vi "fgv_AO_daqmx.vi"(7 "cmd":T1=enum."init", 8 "error in":errorcluster, 11 "level":bool) -> (0 "error out":errorcluster)   [LabVIEW 2019]
uses:
  _ctrl/init-w-close.ctl
  _ctrl/rw.ctl
  SubVIs/common/cmd_err.ctl
  <vilib>/DAQmx/write.llb/DAQmx Write (Analog Wfm 1Chan NSamp).vi
  SubVIs/common/Glob_Ref.vi
  <vilib>/DAQmx/create/channels.llb/DAQmx Create Channel (AO-Voltage-Basic).vi
  <vilib>/DAQmx/configure/timing.llb/DAQmx Timing (Sample Clock).vi
  <vilib>/DAQmx/miscellaneous.llb/DAQmx Fill In Error Info.vi
  Durability/common/Global_params.vi
panel:
  out "task out":refnum<k21>
  out "Waveform Graph":waveform(dbl)(graph)
  out "sample mode":i32(ring)=10178 items=["유한 샘플"=10178, "연속 샘플"=10123, "하드웨어 타이밍에 의한 단일 포인트"=12522]
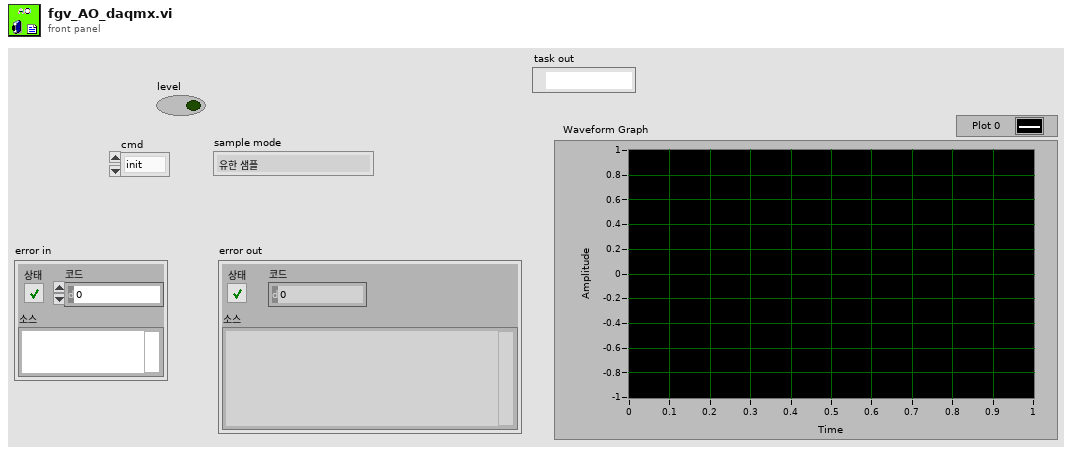
[diagram p1: front panel]
types:
  T1 = typedef "init-w-close.ctl" = enum16{"open", "init", "write", "close"}
  T2 = enum16{"DL950", "BP4610", "DSP1500", "cDAQ-AI", "cDAQ-AO", "cDAQ-DO"}
  T3 = typedef "cmd_err.ctl" = enum16{"close", "open", "default"}
  T4 = typedef "rw.ctl" = enum16{"read", "write"}
  T5 = typedef "cDAQ-9269 Config.ctl" = cluster{"Ch":tag, "Max V":dbl, "Min V":dbl, " Rate":dbl, "N pts":i32, "sample mode":i32}
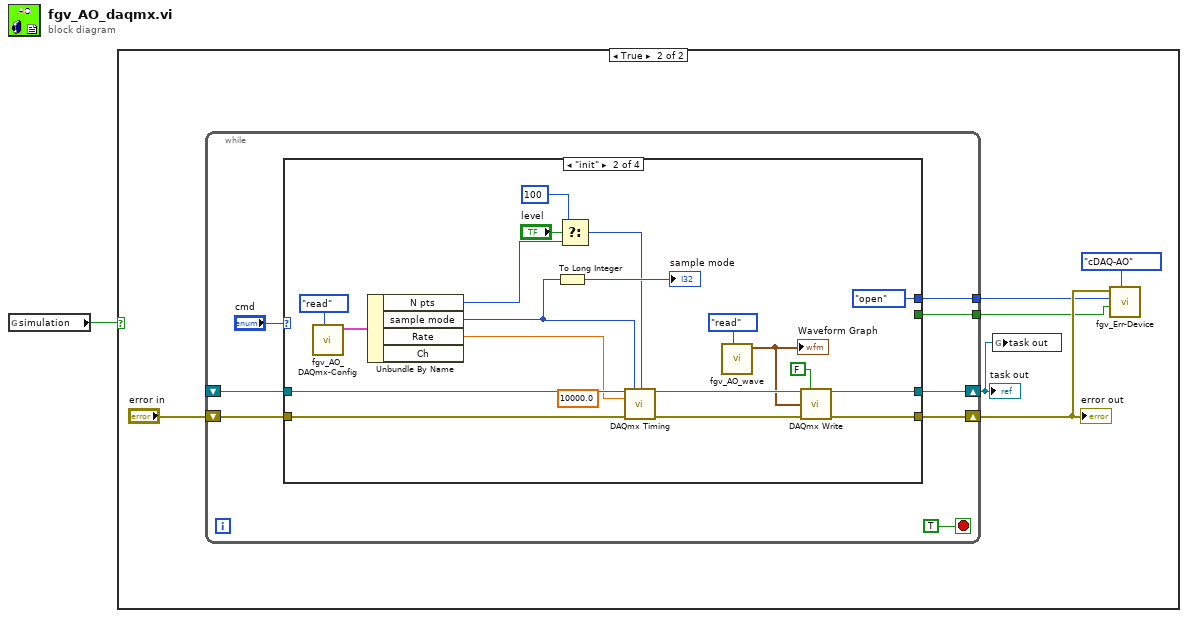
[diagram p0: block diagram]
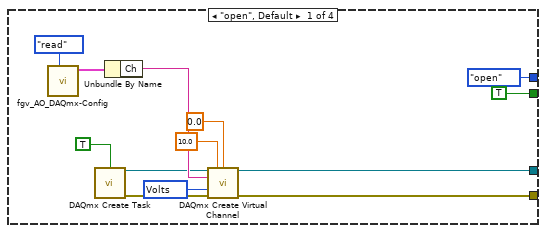
[diagram p3: hidden frame]
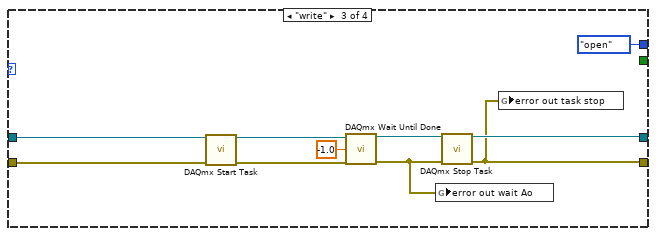
[diagram p4: hidden frame]
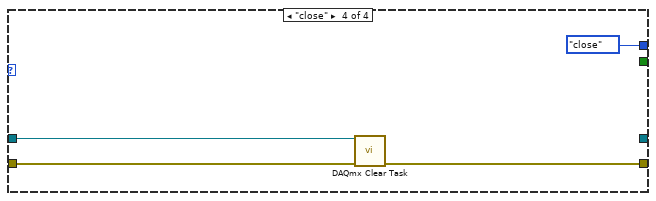
[diagram p5: hidden frame]
diagram:
  n1 = global read "Glob_Ref.vi" "simulation"() -> (w1:bool)
  n2 = case shown="True" w1 {
    frame False {
    }
    frame True {
      n3 = while {
        shift-right: [w13] -> w2
        shift-left: _ -> [w10]
        shift-right: [w12] -> w6
        shift-left: "error in" -> [w11]
        tunnel: [w9] -> w4
        tunnel: [w8] -> w3
        stop <- TRUE stop-if-true
        n4 = case shown="\"init\"" "cmd" {
          tunnel: [w16 w45 w51 _] -> w13
          tunnel: [w22 w46 w48 w59] -> w12
          tunnel: w11 -> [_ w35 w57 w60]
          tunnel: w10 -> [_ w36 w56 w61]
          tunnel: [cmd_err."open" ("cmd") cmd_err."open" ("cmd") cmd_err."open" ("cmd") cmd_err."close" ("cmd")] -> w9
          tunnel: [TRUE ("first?") _ _ _] -> w8
          frame "open", Default {
            w19 = 10348 items=["Volts"=10348, "From Custom Scale"=10065] ("units")
            n5 = call "fgv_AO_DAQmx-Config.vi"("cmd"=rw."read") -> ("config 2"=w27:T5)  [unwired: 9 in, 1 out]
            n6 = call <vilib>:"DAQmx Create Task.vi"("auto cleanup"=TRUE) -> ("task out"=w23:refnum<k21>, "error out"=w24:errorcluster)  [unwired: 13 in]
            n7 = Unbundle By Name(w27) -> ("Ch"=w26:tag)
            n8 = call-poly <vilib>:"DAQmx Create Virtual Channel.vi"("task in"=w23, "maximum value"=10.0, "minimum value"=0.0, "physical channels"=w26, "units"=w19, "error in"=w24) -> ("task out"=w16:refnum<k21>, "error out"=w22:errorcluster)  [unwired: 8 in]
          }
          frame "init" {
            (unwired) 10000.0 ("rate")
            n9 = call "fgv_AO_DAQmx-Config.vi"("cmd"=rw."read") -> ("config 2"=w41:T5)  [unwired: 9 in, 1 out]
            n10 = Unbundle By Name(w41) -> ("N pts"=w32:i32, "sample mode"=w38:i32, "Rate"=w29:dbl)  [unwired: 1 out]
            n11 = To Long Integer(number=w38) -> (32bit integer=→"sample mode":i32)
            n12 = Select(t=100, s="level", f=w32) -> (s? t:f=w31:i32)
            n13 = call-poly <vilib>:"DAQmx Timing.vi"("task/channels in"=w36, "sample mode"=w38, "samples per channel"=w31, "rate"=w29, "error in"=w35) -> ("task out"=w44:refnum<k21>, "error out"=w47:errorcluster)  [unwired: 9 in]
            n14 = call "fgv_AO_wave.vi"("cmd"=rw."read") -> ("signal out"=w37:waveform(dbl))  [unwired: 9 in, 1 out]
            "Waveform Graph" <- w37
            n15 = call-poly <vilib>:"DAQmx Write.vi"("task/channels in"=w44, "auto start"=FALSE, "data"=w37, "error in"=w47) -> ("task out"=w45:refnum<k21>, "error out"=w46:errorcluster)  [unwired: 9 in, 1 out]
          }
          frame "write" {
            n16 = call <vilib>:"DAQmx Start Task.vi"("task/channels in"=w56, "error in"=w57) -> ("task out"=w55:refnum<k21>, "error out"=w53:errorcluster)  [unwired: 12 in]
            n17 = call <vilib>:"DAQmx Wait Until Done.vi"("task/channels in"=w55, "timeout (sec)"=-1.0, "error in"=w53) -> ("task out"=w52:refnum<k21>, "error out"=w49:errorcluster)  [unwired: 11 in]
            n18 = global write "Global_params.vi" "error out wait Ao"(w49) -> ()
            n19 = call <vilib>:"DAQmx Stop Task.vi"("task/channels in"=w52, "error in"=w49) -> ("task out"=w51:refnum<k21>, "error out"=w48:errorcluster)  [unwired: 12 in]
            n20 = global write "Global_params.vi" "error out task stop"(w48) -> ()
          }
          frame "close" {
            n21 = call <vilib>:"DAQmx Clear Task.vi"("task in"=w61, "error in"=w60) -> ("error out"=w59:errorcluster)  [unwired: 13 in]
          }
        }
      }
      "error out" <- w6
      "task out" <- w2
      n22 = global write "Global_params.vi" "task out"(w2) -> ()
      n23 = call "fgv_Err-Device.vi"("Err Sel"=T2."cDAQ-AO", "first?"=w3, "cmd"=w4, "error in"=w6) -> ()  [unwired: 8 in]
    }
  }
